vi "Write data type.vi"(8 "error in (no error)":errorcluster, 10 "data type":dbl, 11 "DSFChannel in":refnum<class "DSFChannel.lvclass">) -> (0 "error out":errorcluster, 3 "DSFChannel out":refnum<class "DSFChannel.lvclass">)   [LabVIEW 2017, in "DSFChannel.lvclass"]
uses:
  DSFChannel.lvclass
  DSFChannel.lvclass/DSFChannel.ctl
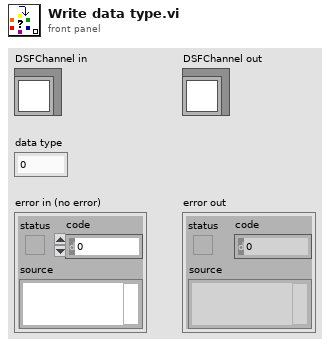
[diagram p1: front panel]
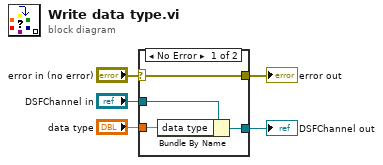
[diagram p0: block diagram]
diagram:
  n1 = case shown="No Error" "error in (no error)" {
    selector: "error in (no error)" -> [w9 w10]
    tunnel: [w9 w10] -> w4
    tunnel: [w7 w11] -> w2
    tunnel: "DSFChannel in" -> [w8 w11]
    tunnel: "data type" -> [w6 _]
    frame No Error {
      n2 = Bundle By Name(cluster=w8, "data type"=w6) -> (w7:refnum<class "DSFChannel.lvclass">)
    }
    frame Error {
    }
  }
  "error out" <- w4
  "DSFChannel out" <- w2
